vi "UpdateChannelMonitorListbox.vi"(8 "error in (no error)":errorcluster, 10 "Monitored Channels":T1[](array[typedef]) {"Data Type" items=["Signed", "Unsigned", "IEEE Float"]}, 11 "Listbox":refnum<vi>) -> (0 "error out":errorcluster)   [LabVIEW 2016, in "LIN Frame Protection Addon System Explorer.lvlib"]
uses:
  LIN Frame Protection Addon System Explorer.lvlib
  Shared/Types/InputChannelConfiguration.ctl
  NationalInstruments.VeriStand
  Shared/LIN Frame Protection Addon Shared.lvlib
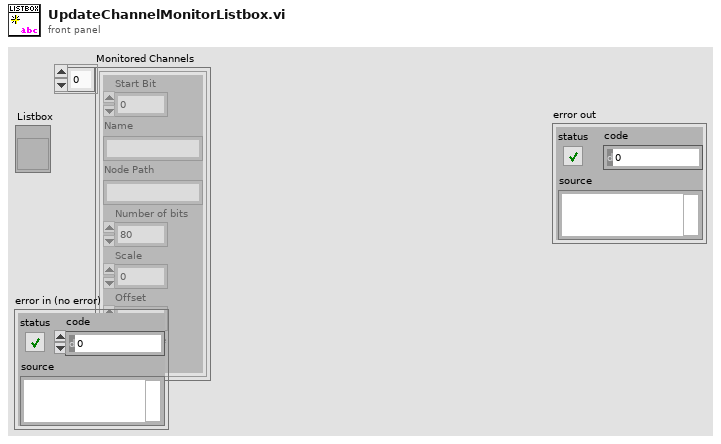
[diagram p1: front panel]
types:
  T1 = typedef "LIN Frame Protection Addon Shared.lvlib/InputChannelConfiguration.ctl" = cluster{"Start Bit":i32, "Name":string, "Node Path":string, "Number of bits":i32, "Scale":dbl, "Offset":dbl, "Data Type":u32}
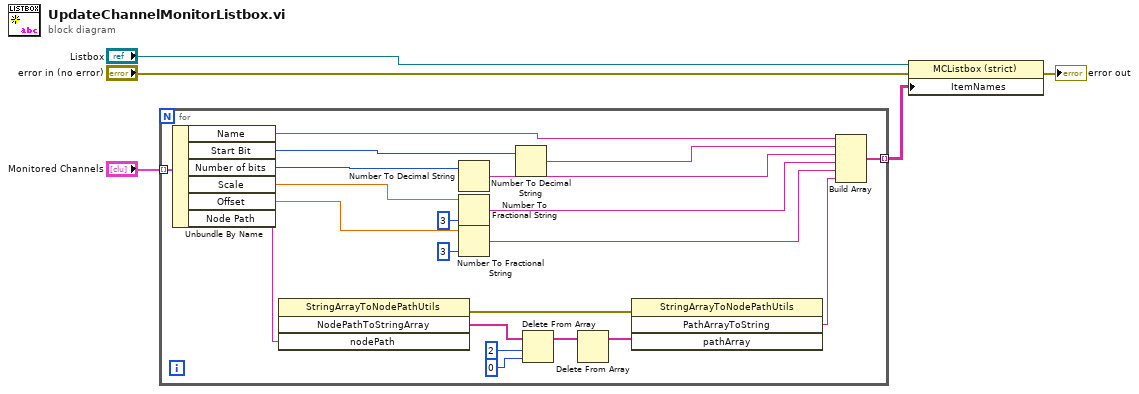
[diagram p0: block diagram]
diagram:
  n1 = for {
    tunnel: "Monitored Channels" -> [w26] mode=indexing
    tunnel: [w16] -> w3 mode=indexing
    n2 = Unbundle By Name(w26) -> ("Name"=w25:string, "Start Bit"=w7:i32, "Number of bits"=w24:i32, "Scale"=w20:dbl, "Offset"=w19:dbl, "Node Path"=w15:string)
    n3 = invoke class="StringArrayToNodePathUtils" method="NodePathToStringArray"("nodePath"=w15) -> (error out=w14:errorcluster, "NodePathToStringArray"=w13:string[])  [unwired: 3 in, 2 out]
    n4 = Number To Decimal String(number=w24) -> (decimal integer string=w23:string)  [unwired: 1 in]
    n5 = Number To Fractional String(number=w20, precision (6)=i16 3) -> (F-format string=w18:string)  [unwired: 2 in]
    n6 = Number To Fractional String(number=w19, precision (6)=i16 3) -> (F-format string=w17:string)  [unwired: 2 in]
    n7 = Number To Decimal String(number=w7) -> (decimal integer string=w6:string)  [unwired: 1 in]
    n8 = Delete From Array(array=w13, length=2, index=0) -> (array with subset deleted=w9:string[])  [unwired: 1 out]
    n9 = Delete From Array(array=w9) -> (array with subset deleted=w8:string[])  [unwired: 2 in, 1 out]
    n10 = invoke class="StringArrayToNodePathUtils" method="PathArrayToString"(error in=w14, "pathArray"=w8) -> ("PathArrayToString"=w10:string)  [unwired: 2 in, 3 out]
    n11 = Build Array(w25, w6, w23, w18, w17, w10) -> (w16:string[])
  }
  n12 = property class="MCListbox (strict)"(reference="Listbox", error in="error in (no error)", "ItemNames"=w3) -> (error out=→"error out":errorcluster)  [unwired: 1 out]
